vi "Find Test Cases in lvlib.vi"(8 "error in (no error)":errorcluster, 11 "Project Path":path) -> (0 "error out":errorcluster, 2 "Test Class paths":path[](array[path]))   [LabVIEW 2020, in "LUnit Test Suite V2.lvclass"]
uses:
  LUnit Test Suite V2.lvclass
  LUnit Test Suite V2.lvclass/LUnit Test Suite V2.ctl
  Utilities/LUnit Utilities.lvlib
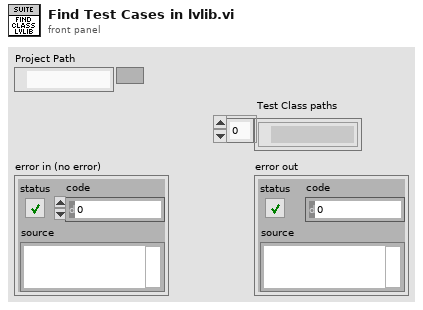
[diagram p1: front panel]
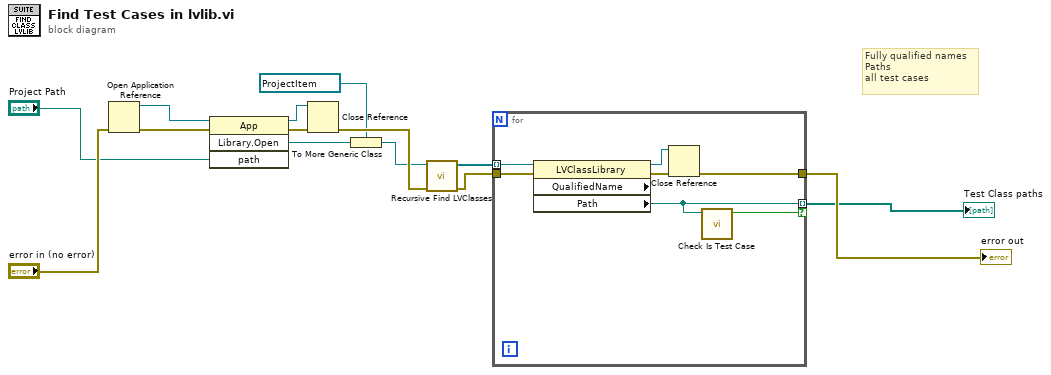
[diagram p0: block diagram]
diagram:
  # "Fully qualified names\nPaths\nall test cases"
  n1 = Open Application Reference(8:"error in (no error)") -> (0:w9:errorcluster, 3:w8:refnum<vi>)  [unwired: 3 in]
  n2 = invoke class="App" method="Library.Open"(reference=w8, error in=w9, "path"="Project Path") -> (reference out=w11:refnum<vi>, error out=w10:errorcluster, "Open Library"=w2:refnum<vi>)  [unwired: 1 in, 1 out]
  n3 = Close Reference(reference=w11, error in (no error)=w10) -> (error out=w4:errorcluster)
  n4 = To More Generic Class(target class=refnum<vi> refnum ("reference"), reference=w2) -> (generic class reference=w1:refnum<vi>)
  n5 = call "Recursive Find LVClasses.vi"("error in (no error)"=w4, "reference"=w1) -> ("error out"=w5:errorcluster, "Class References"=w12:refnum<vi>[])  [unwired: 8 in]
  n6 = for {
    tunnel: w12 -> [w21] mode=indexing
    tunnel: w5 -> [w20]
    tunnel: [w15] -> w14
    tunnel: [w17] -> w6 mode=indexing if=w16
    n7 = property class="LVClassLibrary" props=["QualifiedName", "Path"](reference=w21, error in=w20) -> (reference out=w18:refnum<vi>, error out=w19:errorcluster, "Path"=w17:path)  [unwired: 1 out]
    n8 = Close Reference(reference=w18, error in (no error)=w19) -> (error out=w15:errorcluster)
    n9 = call "Check Is Test Case.vi"("Path"=w17) -> ("Is Test Case?"=w16:bool)  [unwired: 10 in]
  }
  "error out" <- w14
  "Test Class paths" <- w6
